vi "dfd_SCL_SOSIIRIITm_CU.vi"(8 "output valid":bool, 9 "global reset":bool) -> (2 "Control signal":T1)   [LabVIEW 2017]
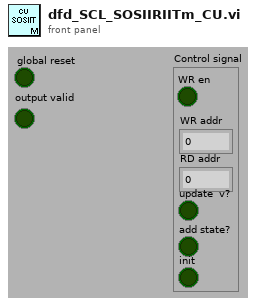
[diagram p1: front panel]
types:
  T1 = cluster{"WR en":bool, "WR addr":u16, "RD addr":u16, "update  v?":bool, "add state?":bool, "init":bool}
  T2 = cluster{"MEM RD Addr":u16, "Ch cnt":u8, "first run?":bool, "MEM Wr Addr":u16}
  T3 = cluster{"circular ctrl(n)":bool, "circular ctrl(n-1)":bool, "circular ctrl(n-2)":bool}
  T4 = cluster{bool, "MEM Wr Addr":u16, "MEM RD Addr":u16, bool, "circular ctrl(n)":bool, bool}
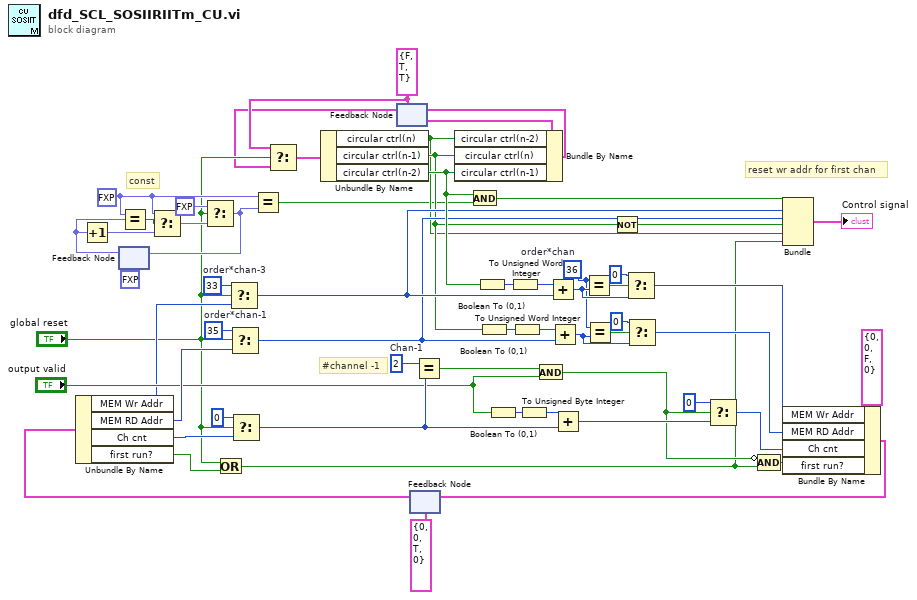
[diagram p0: block diagram]
diagram:
  w10 = fxp<+,3,3> 6.0
  w25 = u16 36  # order*chan
  w37 = u16 33  # order*chan-3
  w5 = T3 {"circular ctrl(n)"=FALSE, "circular ctrl(n-1)"=TRUE, "circular ctrl(n-2)"=TRUE} ("control state out")
  w47 = u8 2  # Chan-1
  w57 = u16 35  # order*chan-1
  # "const"
  # "reset wr addr for first chan"
  # "#channel -1"
  n1 = feedback #1(fxp<+,3,3> 0.0) -> (w13:fxp<+,3,3>)
  n2 = Increment(x=w13) -> (x+1=w12:fxp<+,3,3>)
  n3 = Equal?(x=w10, y=w13) -> (x = y?=w14:bool)
  n4 = Select(t=w10, s=w14, f=w12) -> (s? t:f=w11:fxp<+,3,3>)
  n5 = Select(t=fxp<+,3,3> 1.0, s="global reset", f=w11) -> (s? t:f=w8:fxp<+,3,3>)
  n6 = feedback-in #1(w8) -> ()
  n7 = Equal?(x=w10, y=w8) -> (x = y?=w7:bool)
  n8 = feedback #2(w5) -> (w4:T3)
  n9 = Select(t=w5, s="global reset", f=w4) -> (s? t:f=w3:T3)
  n10 = Unbundle By Name(w3) -> ("circular ctrl(n)"=w17:bool, "circular ctrl(n-1)"=w19:bool, "circular ctrl(n-2)"=w34:bool)
  n11 = feedback #3(T2 {"MEM RD Addr"=0, "Ch cnt"=0, "first run?"=TRUE, "MEM Wr Addr"=0} ("counter state out")) -> (w2:T2)
  n12 = Unbundle By Name(w2) -> ("MEM Wr Addr"=w36:u16, "MEM RD Addr"=w58:u16, "Ch cnt"=w16:u8, "first run?"=w35:bool)
  n13 = Or(x="global reset", y=w35) -> (x .or. y?=w1:bool)
  n14 = Select(t=w37, s="global reset", f=w36) -> (s? t:f=w24:u16)
  n15 = Select(t=w57, s="global reset", f=w58) -> (s? t:f=w23:u16)
  n16 = Select(t=u8 0, s="global reset", f=w16) -> (s? t:f=w46:u8)
  n17 = Equal?(x=w47, y=w46) -> (x = y?=w52:bool)
  n18 = Bundle By Name(cluster=w5, "circular ctrl(n-2)"=w17, "circular ctrl(n)"=w19, "circular ctrl(n-1)"=w34) -> (w42:T3)
  n19 = feedback-in #2(w42) -> ()
  n20 = And(x=w34, y=w7) -> (x .and. y?=w33:bool)
  n21 = Boolean To (0,1)(Boolean=w34) -> (0, 1=w41:i16)
  n22 = Boolean To (0,1)(Boolean=w19) -> (0, 1=w55:i16)
  n23 = Boolean To (0,1)(Boolean="output valid") -> (0, 1=w54:i16)
  n24 = To Unsigned Word Integer(number=w41) -> (unsigned 16bit integer=w40:u16)
  n25 = To Unsigned Word Integer(number=w55) -> (unsigned 16bit integer=w39:u16)
  n26 = To Unsigned Byte Integer(number=w54) -> (unsigned 8bit integer=w53:u8)
  n27 = And(x=w52, y="output valid") -> (x .and. y?=w38:bool)
  n28 = Add(x=w40, y=w24) -> (x+y=w29:u16)
  n29 = Add(x=w39, y=w23) -> (x+y=w26:u16)
  n30 = Add(x=w53, y=w46) -> (x+y=w51:u8)
  n31 = Equal?(x=w25, y=w29) -> (x = y?=w31:bool)
  n32 = Equal?(x=w25, y=w26) -> (x = y?=w27:bool)
  n33 = Not(x=w19) -> (.not. x?=w18:bool)
  n34 = Select(t=u16 0 ("x"), s=w31, f=w29) -> (s? t:f=w21:u16)
  n35 = Select(t=u16 0 ("x"), s=w27, f=w26) -> (s? t:f=w20:u16)
  n36 = Select(t=u8 0, s=w38, f=w51) -> (s? t:f=w49:u8)
  n37 = Compound Arithmetic op=AND(invert w38, w1) -> (w48:bool)
  n38 = Bundle(w33, "MEM Wr Addr"=w24, "MEM RD Addr"=w23, w18, "circular ctrl(n)"=w17, w1) -> (→"Control signal":T4)  [unwired: 1 out]
  n39 = Bundle By Name(cluster=T2 {"MEM RD Addr"=0, "Ch cnt"=0, "first run?"=FALSE, "MEM Wr Addr"=0} ("counter state out"), "MEM Wr Addr"=w21, "MEM RD Addr"=w20, "Ch cnt"=w49, "first run?"=w48) -> (w44:T2)
  n40 = feedback-in #3(w44) -> ()
